vi "transmitRFID v4 cw_query.vi"() -> ()   [LabVIEW 2015]
uses:
  <instrlib>/niUSRP/niUSRP Write Tx Data (CDB).vi
panel:
  in  "query":bool
  out "RFID Pushed":bool
  out "error out":errorcluster
  in  "Parameters Query":T1 {"Session" items=["S0", "S1", "S2", "S3"]; "Sel" items=["All", "All2", "~SL", "SL"]; "M" items=["M=1", "M=2", "M=4", "M=8"]}
  out "Waveform Magnitude":dbl[](graph)
  out "Loop":i32
  in  "Symbol Rate [Hz]":dbl=500000.0 format="%#_13p"
  in  "Parameters Select":T2={"Target"=7, "Action"=0, "MemBank"=1, "truncate"=FALSE} {"MemBank" items=["00 RFU", "01 EPC", "10 TID", "11 User"]; "Action" items=["000", "001", "010", "011", "100", "101", "110", "111"]; "Target" items=["000 Inventoried (S0)", "001 Inventoried (S1)", "010 Inventoried (S2)", "011 Inventoried (S3)", "100 SL", "101 RFU", "110 RFU", "111 RFU"]}
  in  "Parameters Symbols":T3={"Tari"=8e-06, "PW"=0.5, "factor for \"1\" symbol"=0.5, "RTcal"=2.5, "TRcal"=3.0, "Delimiter"=1.4e-05} {"TRcal" min=1.1 max=3.0 step=0.1; "RTcal" min=2.5 max=3.0 step=0.1; "factor for \"1\" symbol" min=0.5 max=1.0 step=0.1; "PW" min=0.265 max=0.525 step=0.001; "Tari" format="%#_3p"}
  out "coerced IQ rate":dbl=100000.0 format="%#_6p"
  out "carrier frequency":dbl=100000.0 format="%#_6p"
  out "coerced gain":dbl format="%#_6f"
  in  "stop":bool
  in  "IQ rate":dbl=2000000.0 format="%#_6p"
  in  "carrier frequency":dbl=920000000.0 format="%#_6p"
  in  "gain":dbl format="%#_6f"
  in  "tx device names":refnum<k15>="192.168.20.13"
  # "Transmit RFID"
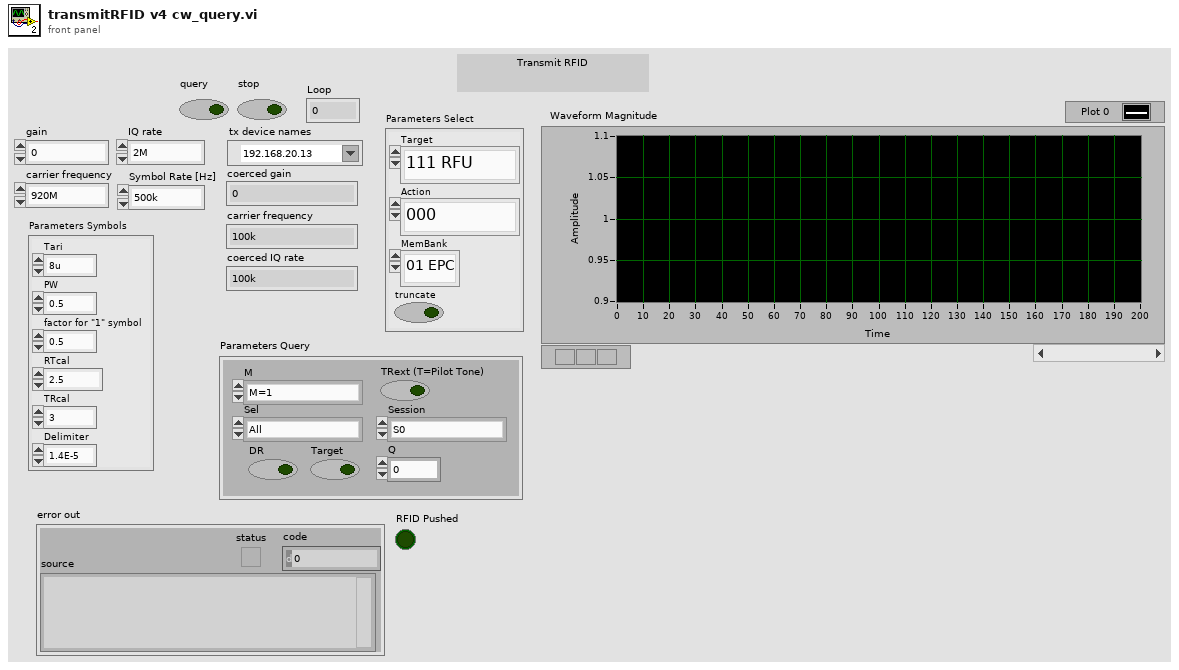
[diagram p1: front panel]
types:
  T1 = cluster{"DR":bool, "M":u16, "TRext (T=Pilot Tone)":bool, "Sel":u16, "Session":u16, "Q":u8, "Target":bool}
  T2 = cluster{"Target":u16, "Action":u16, "MemBank":u16, "truncate":bool}
  T3 = cluster{"Tari":dbl, "PW":dbl, "factor for \"1\" symbol":dbl, "RTcal":dbl, "TRcal":dbl, "Delimiter":dbl}
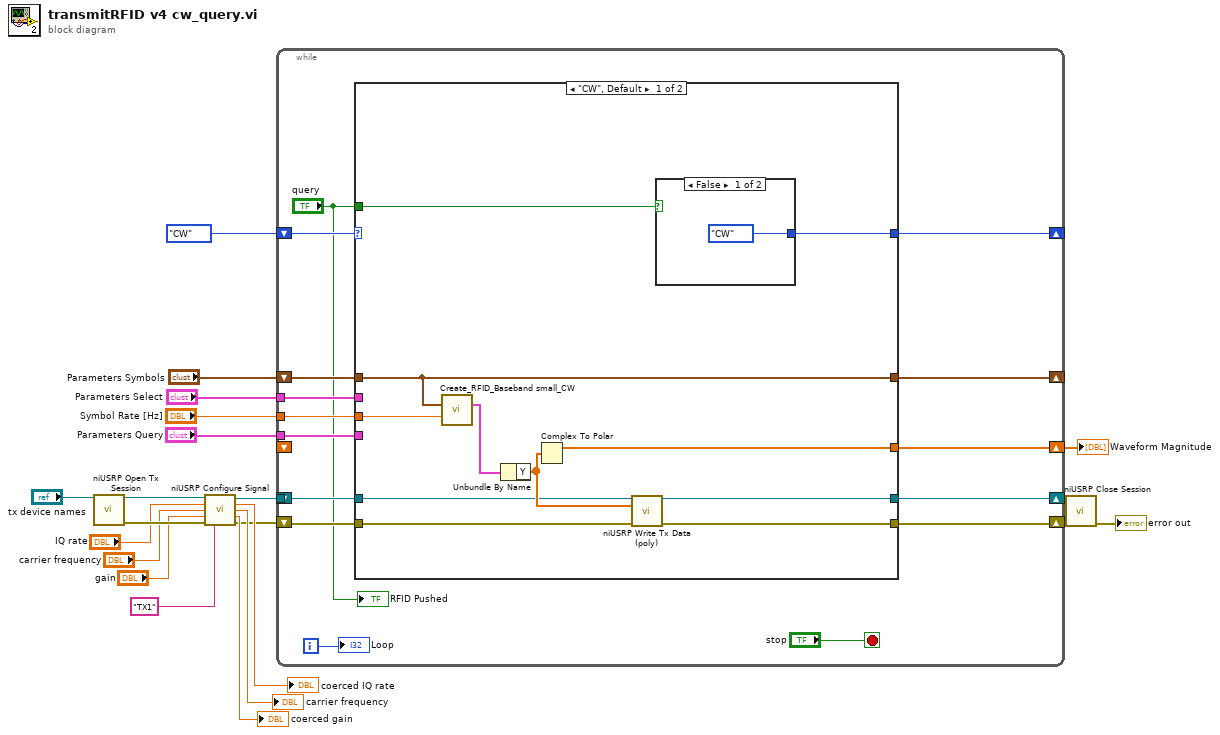
[diagram p0: block diagram]
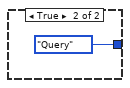
[diagram p2: hidden frame]
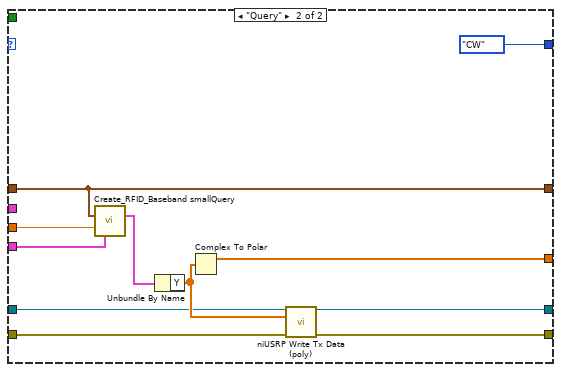
[diagram p3: hidden frame]
diagram:
  n1 = call <instrlib>:"niUSRP Open Tx Session.vi"("device names"="tx device names") -> ("session handle out"=w9:refnum<k15>, "error out"=w21:errorcluster)  [unwired: 13 in]
  n2 = call <instrlib>:"niUSRP Configure Signal.vi"("session handle"=w9, "IQ rate"="IQ rate", "carrier frequency"="carrier frequency", "gain"="gain", "error in (no error)"=w21, "active antenna"="TX1") -> ("session handle out"=w7:refnum<k15>, "coerced IQ rate"=→"coerced IQ rate":dbl, "coerced carrier frequency"=→"carrier frequency":dbl, "coerced gain"=→"coerced gain":dbl, "error out"=w6:errorcluster)  [unwired: 5 in]
  n3 = while {
    tunnel: "Parameters Select" -> [w29]
    tunnel: "Parameters Query" -> [w27]
    tunnel: w7 -> [w34]
    shift-right: [w32] -> w5
    shift-left: w6 -> [w33]
    shift-right: [w31] -> w3
    shift-left: _ -> [_]
    shift-right: [w23] -> _
    shift-left: enum16{"CW", "Query"}."CW" -> [w35]
    shift-right: [w26] -> _
    shift-left: "Parameters Symbols" -> [w30]
    shift-right: [w24] -> w1
    shift-left: _ -> [_]
    tunnel: "Symbol Rate [Hz]" -> [w28]
    i -> [w36]
    stop <- "stop" stop-if-true
    n4 = case shown="\"CW\", Default" w35 {
      tunnel: w34 -> [w46 w59]
      tunnel: w33 -> [w45 w58]
      tunnel: [w44 w57] -> w32
      tunnel: [w43 w56] -> w31
      tunnel: w30 -> [w41 w50]
      tunnel: w29 -> [_ _]
      tunnel: w28 -> [w40 w51]
      tunnel: w27 -> [_ w52]
      tunnel: [w41 w50] -> w26
      tunnel: [w42 w55] -> w24
      tunnel: [w38 enum16{"CW", "Query"}."CW"] -> w23
      tunnel: "query" -> [w37 _]
      frame "CW", Default {
        n5 = call "Create_RFID_Baseband small_CW.vi"("Parameters Symbols"=w41, "Symbol Rate [Hz]"=w40) -> ("complex waveform"=w39:cluster{"t0":dbl, "dt":dbl, "Y":cdb[]})  [unwired: 12 in, 1 out]
        n6 = Unbundle By Name(w39) -> ("Y"=w47:cdb[])
        n7 = Complex To Polar(r * e^(i*theta)=w47) -> (r=w42:dbl[])  [unwired: 1 out]
        n8 = call-poly <instrlib>:"niUSRP Write Tx Data (poly).vi"("session handle"=w46, "data"=w47, "error in (no error)"=w45) -> ("session handle out"=w43:refnum<k15>, "error out"=w44:errorcluster)  [unwired: 11 in]
        n9 = case shown="False" w37 {
          tunnel: [enum16{"CW", "Query"}."CW" enum16{"CW", "Query"}."Query"] -> w38
          frame False {
          }
          frame True {
          }
        }
      }
      frame "Query" {
        n10 = call "Create_RFID_Baseband smallQuery.vi"("Parameters Symbols"=w50, "Symbol Rate [Hz]"=w51, "Parameters Query"=w52) -> ("complex waveform"=w53:cluster{"t0":dbl, "dt":dbl, "Y":cdb[]})  [unwired: 11 in, 1 out]
        n11 = Unbundle By Name(w53) -> ("Y"=w60:cdb[])
        n12 = Complex To Polar(r * e^(i*theta)=w60) -> (r=w55:dbl[])  [unwired: 1 out]
        n13 = call-poly <instrlib>:"niUSRP Write Tx Data (poly).vi"("session handle"=w59, "data"=w60, "error in (no error)"=w58) -> ("session handle out"=w56:refnum<k15>, "error out"=w57:errorcluster)  [unwired: 11 in]
      }
    }
    "Loop" <- w36
    "RFID Pushed" <- "query"
  }
  "Waveform Magnitude" <- w1
  n14 = call <instrlib>:"niUSRP Close Session.vi"("session handle"=w3, "error in (no error)"=w5) -> ("error out"=→"error out":errorcluster)  [unwired: 13 in]
